vi "RDS Child Receive Message.vi"(8 "error in (no error)":errorcluster, 10 "RDS Message":refnum<class "RDS Message.lvclass">, 11 "RDS Mission Controller Actor in":refnum<class "RDS Mission Controller Actor.lvclass">) -> (0 "error out":errorcluster, 3 "RDS Mission Controller Actor out":refnum<class "RDS Mission Controller Actor.lvclass">)   [LabVIEW 2015, in "RDS Mission Controller Actor.lvlib" / "RDS Mission Controller Actor.lvclass"]
uses:
  RDS Mission Controller Actor.lvclass
  Libraries/RDS Framework/RDS Message Class/RDS Message.lvclass
  Libraries/RDS Framework/RDS Message Class/RDS Message.lvclass/RDS Message.ctl
  Libraries/RDS Child Messages/Controller Message/Controller Message.lvclass
  Libraries/RDS Child Messages/Controller Message/Controller Message.lvclass/Controller Message.ctl
  RDS Mission Controller Actor.lvclass/RDS Mission Controller Actor.ctl
  Libraries/RDS Child Messages/Mission Messages/Mission Upload Message.lvclass
  Libraries/RDS Child Messages/Mission Messages/Mission Upload Message.lvclass/Mission Upload Message.ctl
  Libraries/RDS Child Messages/Mission Messages/Mission Set Op Index and Run Msg.lvclass
  Libraries/RDS Child Messages/Mission Messages/Mission Set Op Index and Run Msg.lvclass/Mission Set Op Index and Run Msg.ctl
  Libraries/RDS Child Messages/Controller Message/Controller Message Type.ctl
  Libraries/RDS Child Messages/Mission Messages/Set Mission Controller Settings Message.lvclass
  Libraries/RDS Child Messages/Mission Messages/Set Mission Controller Settings Message.lvclass/Set Mission Controller Settings Message.ctl
  Libraries/RDS Child Messages/GPS Data Message/GPS Data Message.lvclass
  Libraries/RDS Child Messages/GPS Data Message/GPS Data Message.lvclass/GPS Data Message.ctl
  Libraries/RDS Child Messages/Compass/Compass Data Message.lvclass
  Libraries/RDS Child Messages/Compass/Compass Data Message.lvclass/Compass Data Message.ctl
  Actors/RDS Controller Actor/RDS Controller Actor/RDS Controller Actor.lvlib
  Actors/RDS Parent Actor/RDS Parent Actor/RDS Parent Actor.lvclass
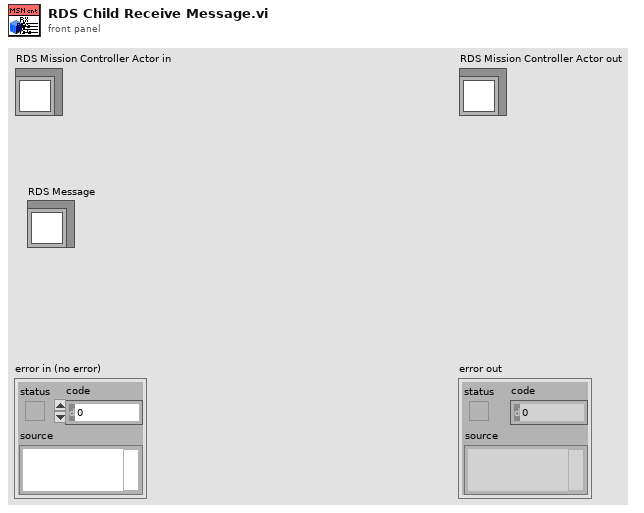
[diagram p1: front panel]
types:
  T1 = typedef "RDS Child Messages.lvlib/Controller Message.lvclass/Controller Message Type.ctl" = enum16{"Control Relinquish Request", "Control Relinquish Command", "Control Request", "Control Granted"}
  T2 = typedef "RDS Child Messages.lvlib/RDS Message ID.ctl" = enum16{"RDS Hello World", "String Message", "AIP_Status", "AIP_Command", "GPS_Data", "MCB_Command", "MCB_Status", "Compass_Data", "Depth_Data", "Battery_Data", "Contoller_State", "Set_Mag_Dev", "BTB_Shutdown", "State_Sample_Request", "State_Sample", "PID_Gains_Set", "Helm_Limiter_Set", "Helm_Heading_Command", "Helm_Steering_Command", "Helm_Status", "Controller_Message", "AIP_Set_Min_Depth", "Mission_Controller_State", "Mission_Upload", "Mission_Set_Op_and_Run", "Mission_Settings_Set"}
  T3 = typedef "RDS Controller Actor.lvlib/Controller.ctl" = enum16{"Idle", "Local Remote Control", "Shore Remote Control", "Mission Control"}
  T4 = typedef "RDS Mission Controller Actor.lvlib/MissionOp.ctl" = cluster{"MissionOp Type":enum16{"Waypoint", "Loiter", "Wait", "Deploy AIP", "Stow AIP"}, "Duration (s)":u16, "Throttle":i16, "GPS Latitude":dbl, "GPS Longitude":dbl, "Loiter Range (m)":u16}
  T5 = typedef "RDS Mission Controller Actor.lvlib/Mission Controller Settings.ctl" = cluster{"Waypoint Radius (m)":dbl}
  T6 = typedef "RDS Libraries.lvlib/NMEA.lvlib/NMEA_GPRMC-data.ctl" = cluster{"TimeStamp":timestamp, "Validity":bool, "Latitude":dbl, "Latitude-Direction":T7, "Longitude":dbl, "Longitude-Direction":T8, "Speed in knots":sgl, "True course":sgl, "Date Stamp":timestamp, "Magnetic Variation (East/West)":sgl, "GPS Latitude":dbl, "GPS Longitude":dbl}
  T7 = typedef "RDS Libraries.lvlib/NMEA.lvlib/NMEA_LatitudeDirection.ctl" = enum16{"", "North", "South"}
  T8 = typedef "RDS Libraries.lvlib/NMEA.lvlib/NMEA_LongitudeDirection.ctl" = enum16{"", "East", "West"}
  T9 = typedef "RDS Instrument Library.lvlib/Compass Data.ctl" = cluster{"Compass Heading":sgl, "pitch Angle":sgl, "roll Angle":sgl, "Temperature":sgl, "Depth":sgl, "Magnetic Field":sgl, "Magnetic Field X":sgl, "Magnetic Field Y":sgl, "Magnetic Field Z":sgl, "Acceleration":sgl, "Acceleration X":sgl, "Acceleration Y":sgl, "Gyro":sgl, "Gyro X":sgl, "Acceleration Z":sgl, "Gyro Y":sgl, "Raw Heading":sgl}
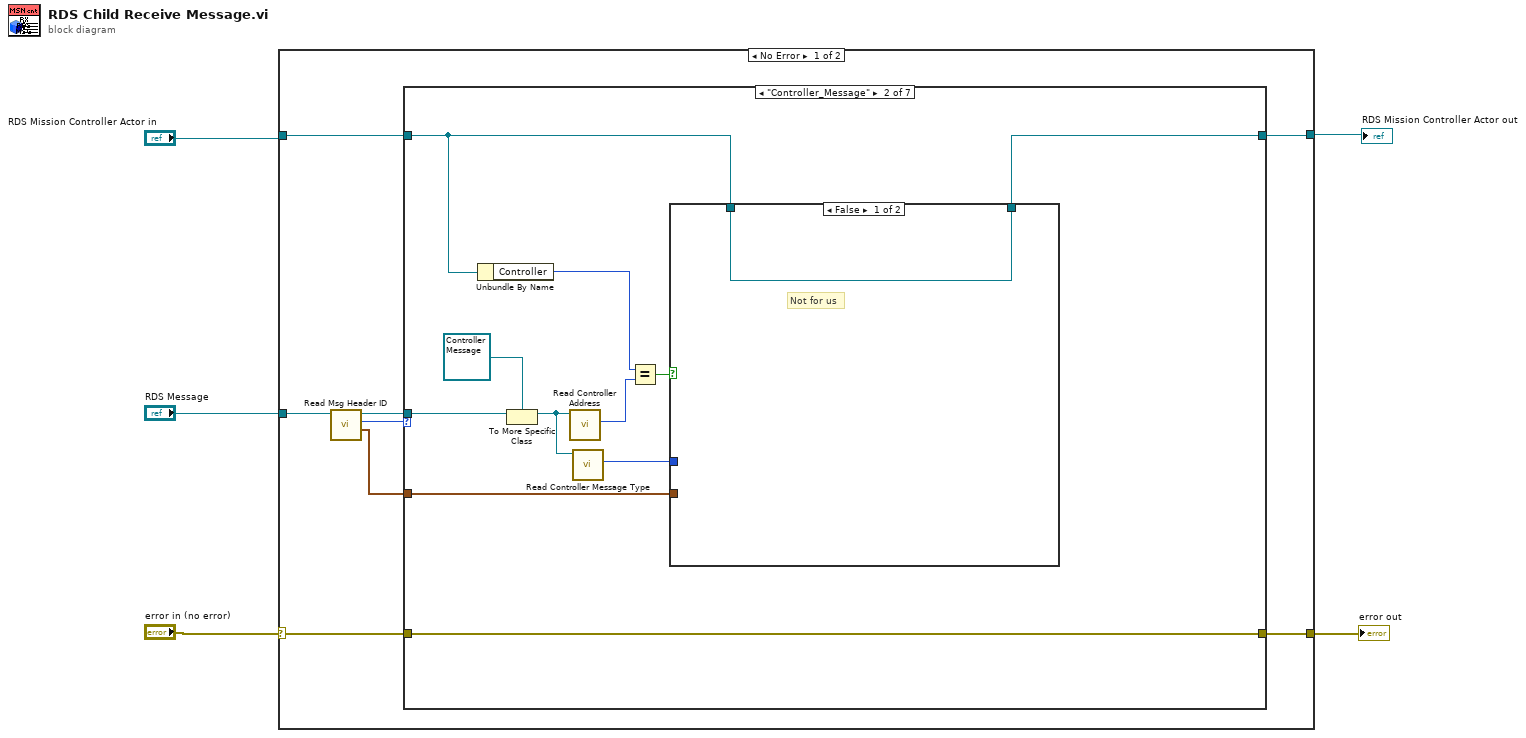
[diagram p0: block diagram]
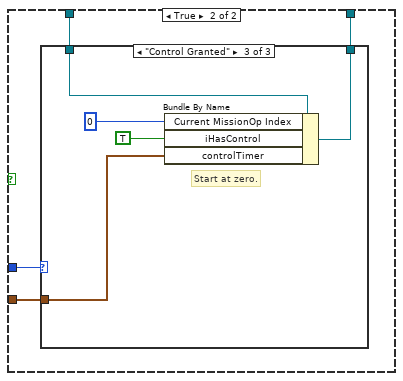
[diagram p3: hidden frame]
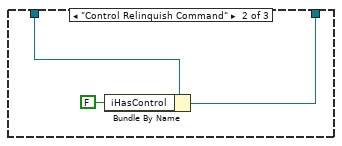
[diagram p5: hidden frame]
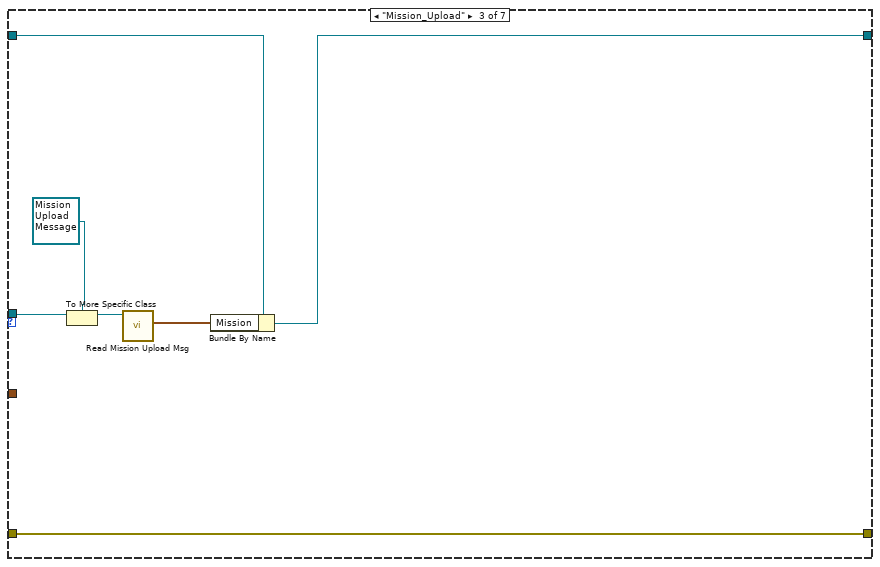
[diagram p6: hidden frame]
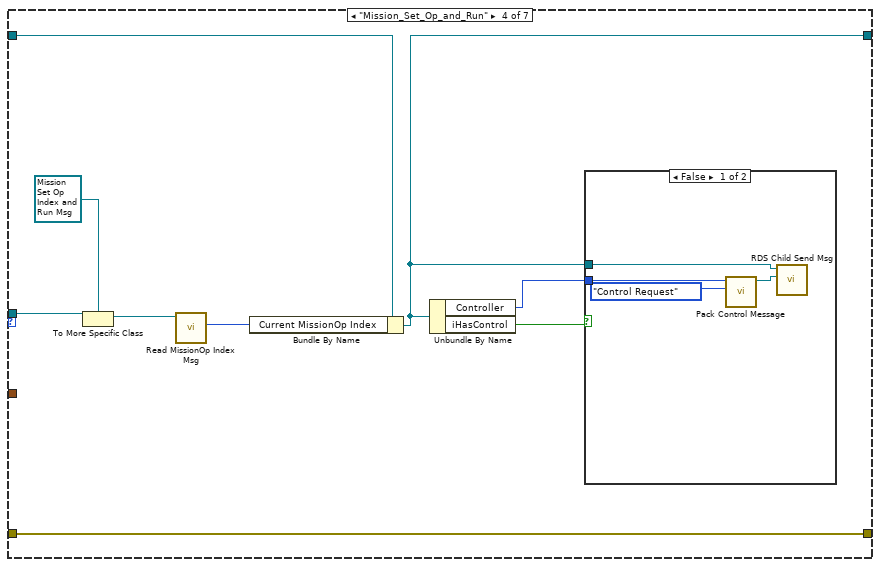
[diagram p7: hidden frame]
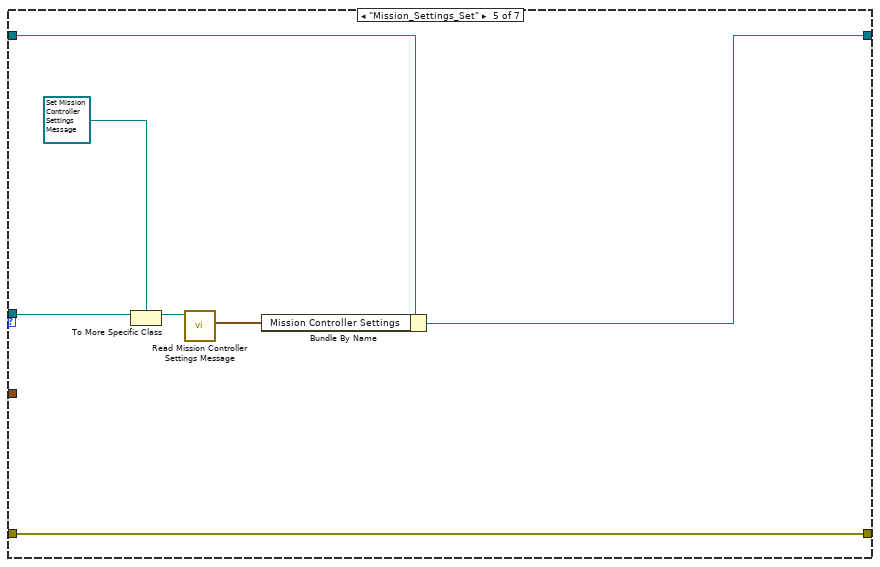
[diagram p9: hidden frame]
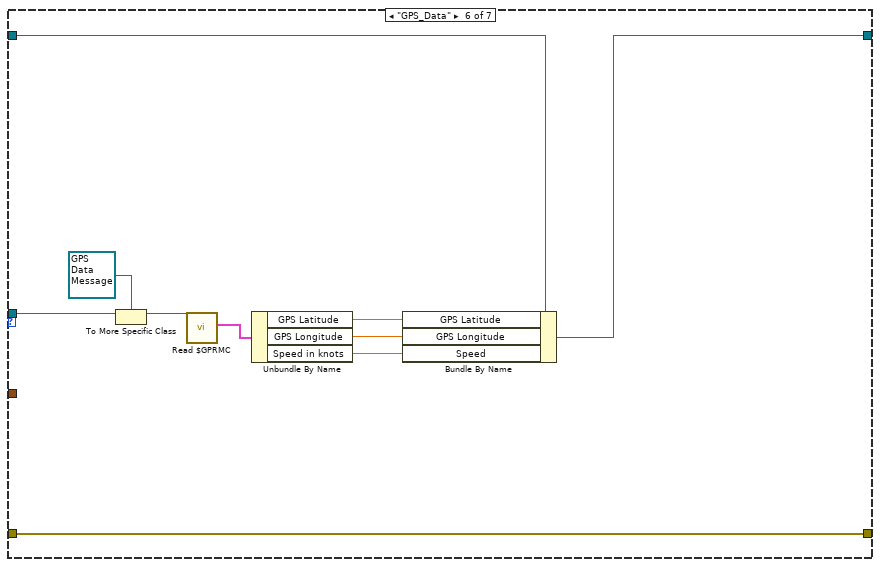
[diagram p10: hidden frame]
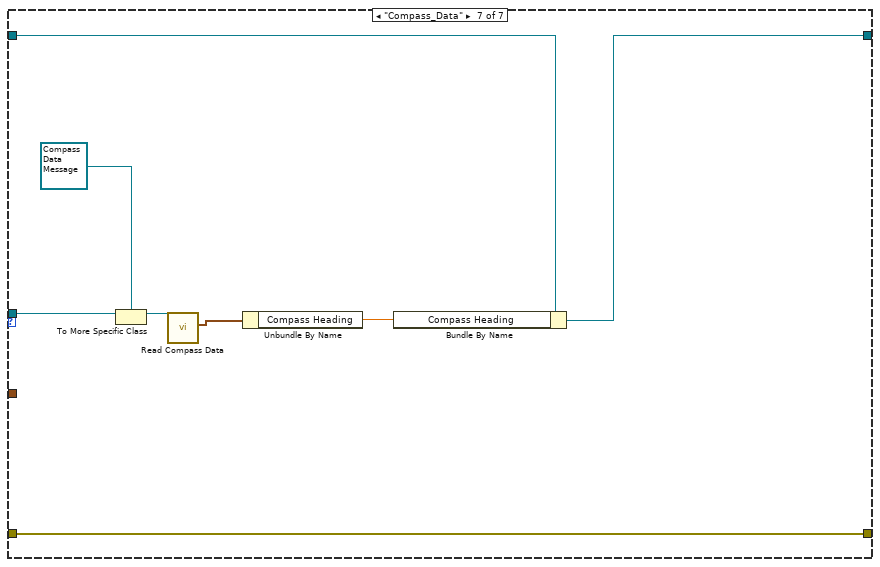
[diagram p11: hidden frame]
diagram:
  n1 = case shown="No Error" "error in (no error)" {
    selector: "error in (no error)" -> [w9 w86]
    tunnel: "RDS Message" -> [w13 _]
    tunnel: "RDS Mission Controller Actor in" -> [w7 w87]
    tunnel: [w8 w87] -> w2
    tunnel: [w10 w86] -> w1
    frame No Error {
      n2 = call "Read Msg Header ID.vi"("RDS Message in"=w13) -> ("Time Stamp"=w6:timestamp, "Msg ID"=w12:T2, "RDS Message out"=w11:refnum<class "RDS Message.lvclass">)  [unwired: 6 in, 2 out]
      n3 = case shown="\"Controller_Message\"" w12 {
        tunnel: w11 -> [_ w26 w46 w55 w66 w75 w84]
        tunnel: [w15 w25 w47 w56 w67 w77 w85] -> w10
        tunnel: w9 -> [w15 w25 w47 w56 w67 w77 w85]
        tunnel: w7 -> [w14 w19 w42 w51 w65 w69 w82]
        tunnel: [w14 w21 w41 w49 w64 w68 w81] -> w8
        tunnel: w6 -> [_ w20 _ _ _ _ _]
        frame "RDS Hello World", Default {
        }
        frame "Controller_Message" {
          n4 = Unbundle By Name(w19) -> ("Controller"=w17:T3)
          n5 = To More Specific Class(target class=refnum<class "Controller Message.lvclass"> refnum ("RDS Child Messages.lvlib:Controller Message.lvclass"), reference=w26) -> (specific class reference=w23:refnum<class "Controller Message.lvclass">)  [unwired: 1 in, 1 out]
          n6 = call "Read Controller Address.vi"("Controller Message in"=w23) -> ("Controller"=w18:T3)  [unwired: 8 in, 2 out]
          n7 = call "Read Controller Message Type.vi"("Controller Message in"=w23) -> ("Controller Message Type"=w22:T1)  [unwired: 8 in, 2 out]
          n8 = Equal?(x=w17, y=w18) -> (x = y?=w16:bool)
          n9 = case shown="False" w16 {
            tunnel: w22 -> [_ w31]
            tunnel: w19 -> [w27 w30]
            tunnel: [w27 w29] -> w21
            tunnel: w20 -> [_ w28]
            frame False {
              # "Not for us"
            }
            frame True {
              n10 = case shown="\"Control Granted\"" w31 {
                tunnel: w30 -> [w32 w35 w40]
                tunnel: [w32 w33 w38] -> w29
                tunnel: w28 -> [_ _ w37]
                frame "Control Relinquish Request", Default {
                  # "not for us"
                }
                frame "Control Relinquish Command" {
                  n11 = Bundle By Name(cluster=w35, "iHasControl"=FALSE) -> (w33:refnum<class "RDS Mission Controller Actor.lvclass">)
                }
                frame "Control Granted" {
                  # "Start at zero."
                  n12 = Bundle By Name(cluster=w40, "Current MissionOp Index"=0, "iHasControl"=TRUE, "controlTimer"=w37) -> (w38:refnum<class "RDS Mission Controller Actor.lvclass">)
                }
              }
            }
          }
        }
        frame "Mission_Upload" {
          n13 = To More Specific Class(target class=refnum<class "Mission Upload Message.lvclass"> refnum ("RDS Child Messages.lvlib:Load Mission Message.lvclass"), reference=w46) -> (specific class reference=w44:refnum<class "Mission Upload Message.lvclass">)  [unwired: 1 in, 1 out]
          n14 = call "Read Mission Upload Msg.vi"("Load Mission Message in"=w44) -> ("Mission"=w43:T4[])  [unwired: 8 in, 2 out]
          n15 = Bundle By Name(cluster=w42, "Mission"=w43) -> (w41:refnum<class "RDS Mission Controller Actor.lvclass">)
        }
        frame "Mission_Set_Op_and_Run" {
          n16 = To More Specific Class(target class=refnum<class "Mission Set Op Index and Run Msg.lvclass"> refnum ("RDS Child Messages.lvlib:Mission Set Op Index and Run Msg.lvclass"), reference=w55) -> (specific class reference=w53:refnum<class "Mission Set Op Index and Run Msg.lvclass">)  [unwired: 1 in, 1 out]
          n17 = call "Read MissionOp Index Msg.vi"("Mission Set Op Index and Run Msg in"=w53) -> ("MissionOp Index"=w52:i32)  [unwired: 8 in, 2 out]
          n18 = Bundle By Name(cluster=w51, "Current MissionOp Index"=w52) -> (w49:refnum<class "RDS Mission Controller Actor.lvclass">)
          n19 = Unbundle By Name(w49) -> ("Controller"=w48:T3, "iHasControl"=w50:bool)
          n20 = case shown="False" w50 {
            tunnel: w49 -> [w57 _]
            tunnel: w48 -> [w60 _]
            frame False {
              n21 = call "Pack Control Message.vi"("Controller Message Type"=Controller_Message_Type."Control Request", "Controller"=w60) -> ("Controller Message out"=w58:refnum<class "Controller Message.lvclass">)  [unwired: 9 in]
              n22 = call "RDS Child Send Msg.vi"("RDS Message"=w58, "RDS Parent Actor in"=w57) -> ()  [unwired: 8 in, 2 out]
            }
            frame True {
            }
          }
        }
        frame "Mission_Settings_Set" {
          n23 = To More Specific Class(target class=refnum<class "Set Mission Controller Settings Message.lvclass"> refnum ("RDS Child Messages.lvlib:Set Mission Controller Settings Message.lvclass"), reference=w66) -> (specific class reference=w62:refnum<class "Set Mission Controller Settings Message.lvclass">)  [unwired: 1 in, 1 out]
          n24 = call "Read Mission Controller Settings Message.vi"("Set Mission Controller Settings Message in"=w62) -> ("Mission Controller Settings"=w61:T5)  [unwired: 8 in, 2 out]
          n25 = Bundle By Name(cluster=w65, "Mission Controller Settings"=w61) -> (w64:refnum<class "RDS Mission Controller Actor.lvclass">)
        }
        frame "GPS_Data" {
          n26 = To More Specific Class(target class=refnum<class "GPS Data Message.lvclass"> refnum ("RDS Child Messages.lvlib:GPS Data Message.lvclass"), reference=w75) -> (specific class reference=w76:refnum<class "GPS Data Message.lvclass">)  [unwired: 1 in, 1 out]
          n27 = call "Read $GPRMC.vi"("GPS Data Message in"=w76) -> ("GPRMC-data"=w73:T6)  [unwired: 8 in, 2 out]
          n28 = Unbundle By Name(w73) -> ("GPS Latitude"=w70:dbl, "GPS Longitude"=w71:dbl, "Speed in knots"=w72:sgl)
          n29 = Bundle By Name(cluster=w69, "GPS Latitude"=w70, "GPS Longitude"=w71, "Speed"=w72) -> (w68:refnum<class "RDS Mission Controller Actor.lvclass">)
        }
        frame "Compass_Data" {
          n30 = To More Specific Class(target class=refnum<class "Compass Data Message.lvclass"> refnum ("RDS Child Messages.lvlib:Compass Data Message.lvclass"), reference=w84) -> (specific class reference=w79:refnum<class "Compass Data Message.lvclass">)  [unwired: 1 in, 1 out]
          n31 = call "Read Compass Data.vi"("Compass Data Message in"=w79) -> ("Compass Data"=w78:T9)  [unwired: 8 in, 2 out]
          n32 = Unbundle By Name(w78) -> ("Compass Heading"=w83:sgl)
          n33 = Bundle By Name(cluster=w82, "Compass Heading"=w83) -> (w81:refnum<class "RDS Mission Controller Actor.lvclass">)
        }
      }
    }
    frame Error {
    }
  }
  "error out" <- w1
  "RDS Mission Controller Actor out" <- w2
